vi "new_NeuralNetwork.vi"() -> ()   [LabVIEW 2014]
panel:
  out "Weights":dbl[](array[numeric])
  out "appended array 2":dbl[](array[numeric])
  out "appended array":dbl[](array[numeric])
  in  "Mode":enum16{"Forward Pass", "Testing"}(ring)
  in  "Axis":enum16{"X", "Y", "Z"}(ring)
  in  "stop":bool
  out "z":dbl
  out "y":dbl
  out "x":dbl
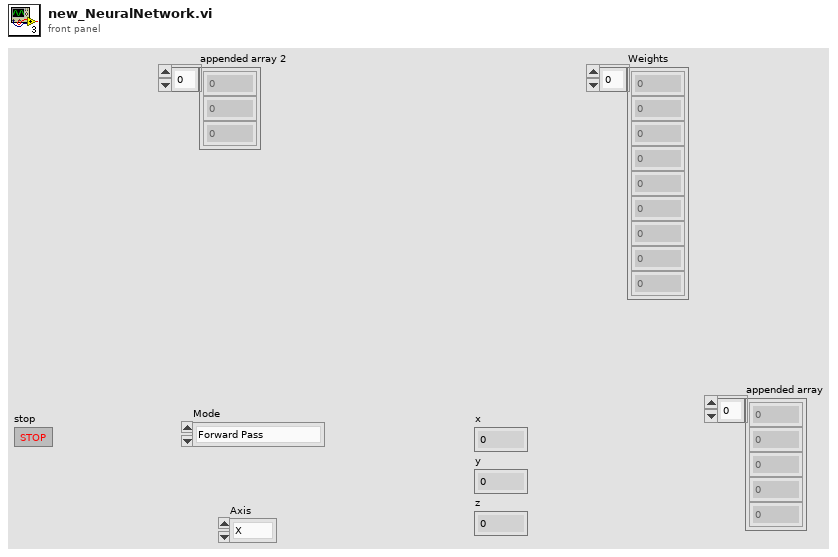
[diagram p1: front panel]
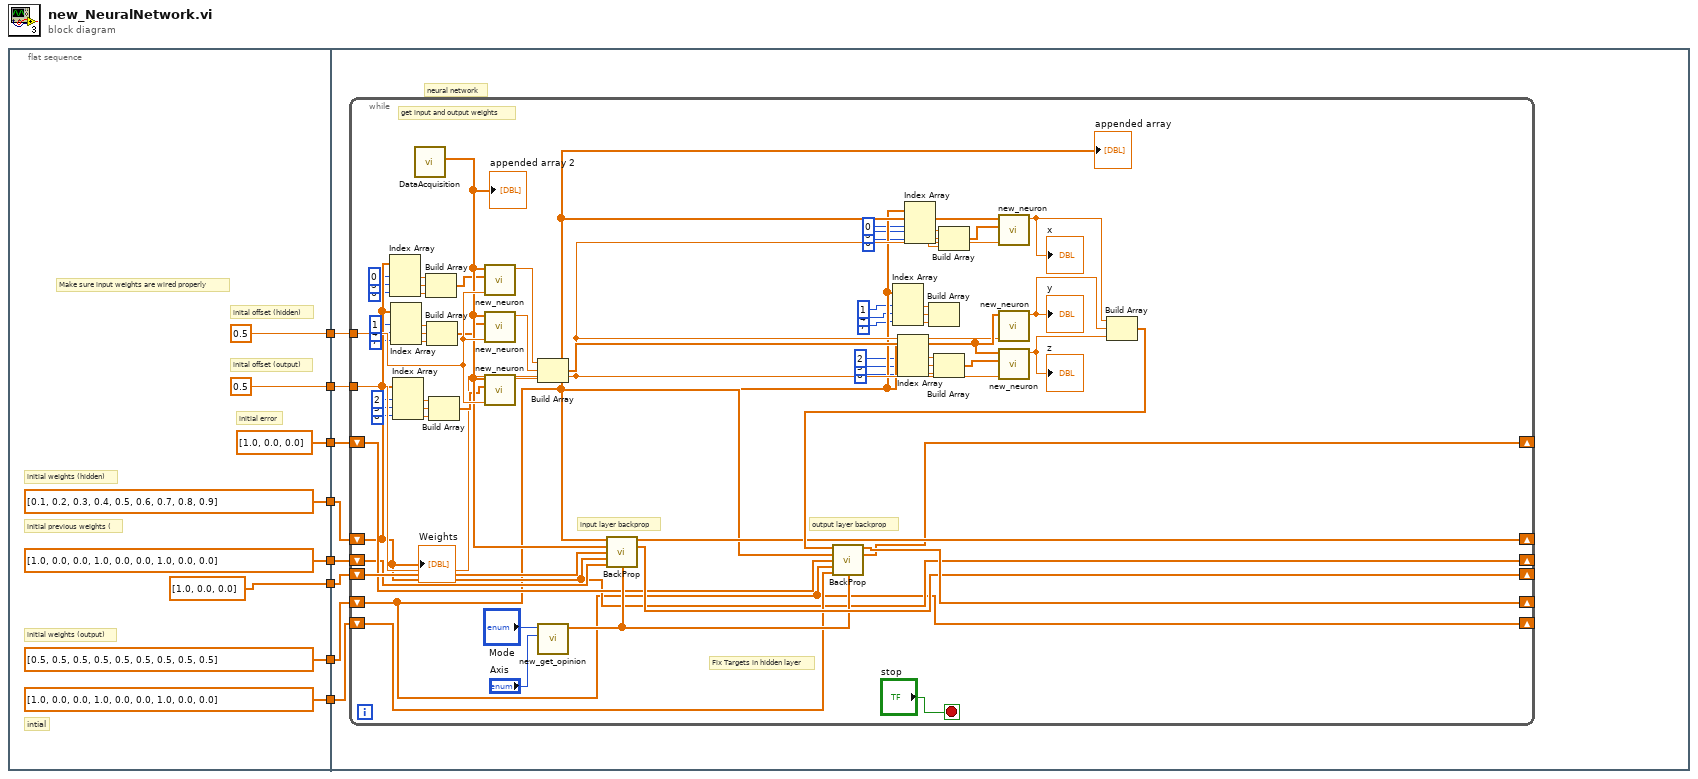
[diagram p0: block diagram]
diagram:
  n1 = flat-sequence {
    tunnel: [0.5] -> w8
    tunnel: [dbl[] [0.1, 0.2, 0.3, 0.4, 0.5, 0.6, 0.7, 0.8, 0.9] ("Weights")] -> w7
    tunnel: [dbl[] [0.5, 0.5, 0.5, 0.5, 0.5, 0.5, 0.5, 0.5, 0.5] ("Weights")] -> w6
    tunnel: [0.5] -> w5
    tunnel: [dbl[] [1.0, 0.0, 0.0] ("dE_dNET")] -> w4
    tunnel: [dbl[] [1.0, 0.0, 0.0, 1.0, 0.0, 0.0, 1.0, 0.0, 0.0] ("Weights")] -> w3
    tunnel: [dbl[] [1.0, 0.0, 0.0, 1.0, 0.0, 0.0, 1.0, 0.0, 0.0] ("Weights")] -> w2
    tunnel: [dbl[] [1.0, 0.0, 0.0] ("dE_dNET")] -> w1
    tunnel: w8 -> [w24]
    tunnel: w7 -> [w23]
    tunnel: w6 -> [w21]
    tunnel: w5 -> [w22]
    tunnel: w4 -> [w19]
    tunnel: w3 -> [w20]
    tunnel: w2 -> [w18]
    tunnel: w1 -> [w17]
    frame #0 {
      # "Make sure input weights are wired properly"
      # "initial previous weights ("
      # "intial"
      # "initial error"
      # "inital offset (output)"
      # "inital offset (hidden)"
      # "initial weights (output)"
      # "initial weights (hidden)"
    }
    frame #1 {
      # "neural network"
      n2 = while {
        tunnel: w24 -> [w88]
        tunnel: w22 -> [w64]
        shift-right: [w70] -> _
        shift-left: w19 -> [w76]
        shift-right: [w85] -> _
        shift-left: w21 -> [w34]
        shift-right: [w84] -> _
        shift-left: w17 -> [w83]
        shift-right: [w34] -> _
        shift-left: w18 -> [w71]
        shift-right: [w73] -> _
        shift-left: w23 -> [w55]
        shift-right: [w55] -> _
        shift-left: w20 -> [w72]
        stop <- "stop" stop-if-true
        # "Fix Targets in hidden layer"
        # "get input and output weights"
        # "output layer backprop"
        # "input layer backprop"
        n3 = Index Array(array=w55, index #1=0 ("index"), index #2=3 ("index"), index #3=6 ("index")) -> (element #1=w60:dbl, element #2=w59:dbl, element #3=w58:dbl)
        n4 = Index Array(array=w55, index #1=1 ("index"), index #2=4 ("index"), index #3=7 ("index")) -> (element #1=w63:dbl, element #2=w62:dbl, element #3=w61:dbl)
        n5 = Index Array(array=w55, index #1=2 ("index"), index #2=5 ("index"), index #3=8 ("index")) -> (element #1=w68:dbl, element #2=w67:dbl, element #3=w66:dbl)
        n6 = call "DataAcquisition.vi"() -> ("appended array"=w74:dbl[])  [unwired: 10 in, 1 out]
        "appended array 2" <- w74
        n7 = Build Array(w60, w59, w58) -> (w57:dbl[])
        n8 = Build Array(w63, w62, w61) -> (w56:dbl[])
        n9 = Build Array(w68, w67, w66) -> (w65:dbl[])
        n10 = call "new_neuron.vi"("Offset"=w88, "Weights"=w57, "Inputs"=w74) -> ("Output"=w90:dbl)  [unwired: 8 in]
        n11 = call "new_neuron.vi"("Offset"=w88, "Weights"=w56, "Inputs"=w74) -> ("Output"=w86:dbl)  [unwired: 8 in]
        n12 = call "new_neuron.vi"("Offset"=w88, "Weights"=w65, "Inputs"=w74) -> ("Output"=w89:dbl)  [unwired: 8 in]
        n13 = Build Array(w90, w86, w89) -> (w69:dbl[])
        "appended array" <- w69
        n14 = call "new_get_opinion.vi"("Axis"="Axis", "Mode"="Mode") -> ("opinons"=w81:dbl[])  [unwired: 9 in]
        n15 = call "BackProp.vi"("Current Layer"=w69, "Previous Layer"=w74, "NetError"=w83, "weights"=w55, "PreviousWeights"=w72, "Target"=w81) -> ("w+"=w73:dbl[], "dE_dNET"=w84:dbl[])  [unwired: 8 in]
        n16 = Index Array(array=w34, index #1=1 ("index"), index #2=4 ("index"), index #3=7 ("index")) -> (element #1=w41:dbl, element #2=w40:dbl, element #3=w39:dbl)
        n17 = Index Array(array=w34, index #1=2 ("index"), index #2=5 ("index"), index #3=8 ("index")) -> (element #1=w45:dbl, element #2=w44:dbl, element #3=w43:dbl)
        n18 = Index Array(array=w34, index #1=0 ("index"), index #2=3 ("index"), index #3=6 ("index")) -> (element #1=w38:dbl, element #2=w37:dbl, element #3=w36:dbl)
        n19 = Build Array(w41, w40, w39) -> ()  [unwired: 1 out]
        n20 = Build Array(w45, w44, w43) -> (w42:dbl[])
        n21 = Build Array(w38, w37, w36) -> (w35:dbl[])
        n22 = call "new_neuron.vi"("Offset"=w64, "Weights"=w35, "Inputs"=w69) -> ("Output"=w80:dbl)  [unwired: 8 in]
        "x" <- w80
        n23 = call "new_neuron.vi"("Offset"=w64, "Inputs"=w69) -> ("Output"=w79:dbl)  [unwired: 9 in]
        "y" <- w79
        n24 = call "new_neuron.vi"("Offset"=w64, "Weights"=w42, "Inputs"=w69) -> ("Output"=w78:dbl)  [unwired: 8 in]
        "z" <- w78
        n25 = Build Array(w80, w79, w78) -> (w77:dbl[])
        n26 = call "BackProp.vi"("Current Layer"=w77, "Previous Layer"=w69, "NetError"=w76, "weights"=w34, "PreviousWeights"=w71, "Target"=w81) -> ("w+"=w85:dbl[], "dE_dNET"=w70:dbl[])  [unwired: 8 in]
        "Weights" <- w55
      }
    }
  }
